vi "GEOM_CalcHeaders.vi"(8 "error in (no error)":errorcluster, 9 "modifiers":T2={"Binning"={"x"=1, "y"=1}, "sections"=[{"name"="", "header section"="", "comment"="", "value"=20, "binning?"=FALSE, "Where"=enum."predata", "add In"=enum."columns"}, {"name"="", "header section"="", "comment"="", "value"=64, "binning?"=FALSE, "Where"=enum."postdata", "add In"=enum."columns"}, {"name"="", "header section"="", "comment"="", "value"=14, "binning?"=FALSE, "Where"=enum."postdata", "add In"=enum."none"}]} {"Binning"."y" min=1; "Binning"."x" min=1}, 10 "FPAReadModes":T5[](array[typedef])=[{"name"="quad", "Amplifiers"=[{"number"=0, "type"=0, "rotated"=0, "fliped"=0, "FPAcoord"={"xstart"=1, "ystart"=1}, "Physical_size"={"columns"=1024, "rows"=1024}, "predata"={"columns"=20, "rows"=0}, "postdata"={"columns"=64, "rows"=0}, "Req ROIs"=[], "Corr ROI"=[], "Detnumber"=0, "ampID"="", "discard"=0}, {"number"=0, "type"=1, "rotated"=0, "fliped"=0, "FPAcoord"={"xstart"=1025, "ystart"=1}, "Physical_size"={"columns"=1024, "rows"=1024}, "predata"={"columns"=20, "rows"=0}, "postdata"={"columns"=64, "rows"=0}, "Req ROIs"=[], "Corr ROI"=[], "Detnumber"=0, "ampID"="", "discard"=0}, {"number"=0, "type"=2, "rotated"=0, "fliped"=0, "FPAcoord"={"xstart"=1, "ystart"=1025}, "Physical_size"={"columns"=1024, "rows"=1024}, "predata"={"columns"=20, "rows"=0}, "postdata"={"columns"=64, "rows"=0}, "Req ROIs"=[], "Corr ROI"=[], "Detnumber"=0, "ampID"="", "discard"=0}, {"number"=0, "type"=3, "rotated"=0, "fliped"=0, "FPAcoord"={"xstart"=1025, "ystart"=1025}, "Physical_size"={"columns"=1024, "rows"=1024}, "predata"={"columns"=20, "rows"=0}, "postdata"={"columns"=64, "rows"=0}, "Req ROIs"=[], "Corr ROI"=[], "Detnumber"=0, "ampID"="", "discard"=0}]}, {"name"="lowerleft", "Amplifiers"=[{"number"=0, "type"=0, "rotated"=0, "fliped"=0, "FPAcoord"={"xstart"=1, "ystart"=1}, "Physical_size"={"columns"=2048, "rows"=2048}, "predata"={"columns"=20, "rows"=0}, "postdata"={"columns"=64, "rows"=0}, "Req ROIs"=[], "Corr ROI"=[], "Detnumber"=0, "ampID"="", "discard"=0}]}] {"Amplifiers"."fliped" items=["none", "horizontal", "vertical"]; "Amplifiers"."type" items=["LL", "LR", "UL", "UR"]}, 11 "moddir":path=path "/kkk") -> (0 "error out":errorcluster)   [LabVIEW 2016]
uses:
  GEOM_FPAReadMode.ctl
  GEOM_Amplifier.ctl
  GEOM_AmpType.ctl
  GEOM_ROI.ctl
  GEOM_Coords.ctl
  GEOM_AmpModifiers.ctl
  GEOM_Binning.ctl
  GEOM_Moifier.ctl
  GEOM_ReadModeHeader.ctl
  GEOM_VAR_action.ctl
panel:
  in  "type specifier VI Refnum (for type only)":refnum<vi>
  in  "Empty Array 2":string[][](array[string])
  in  "Headers":T1
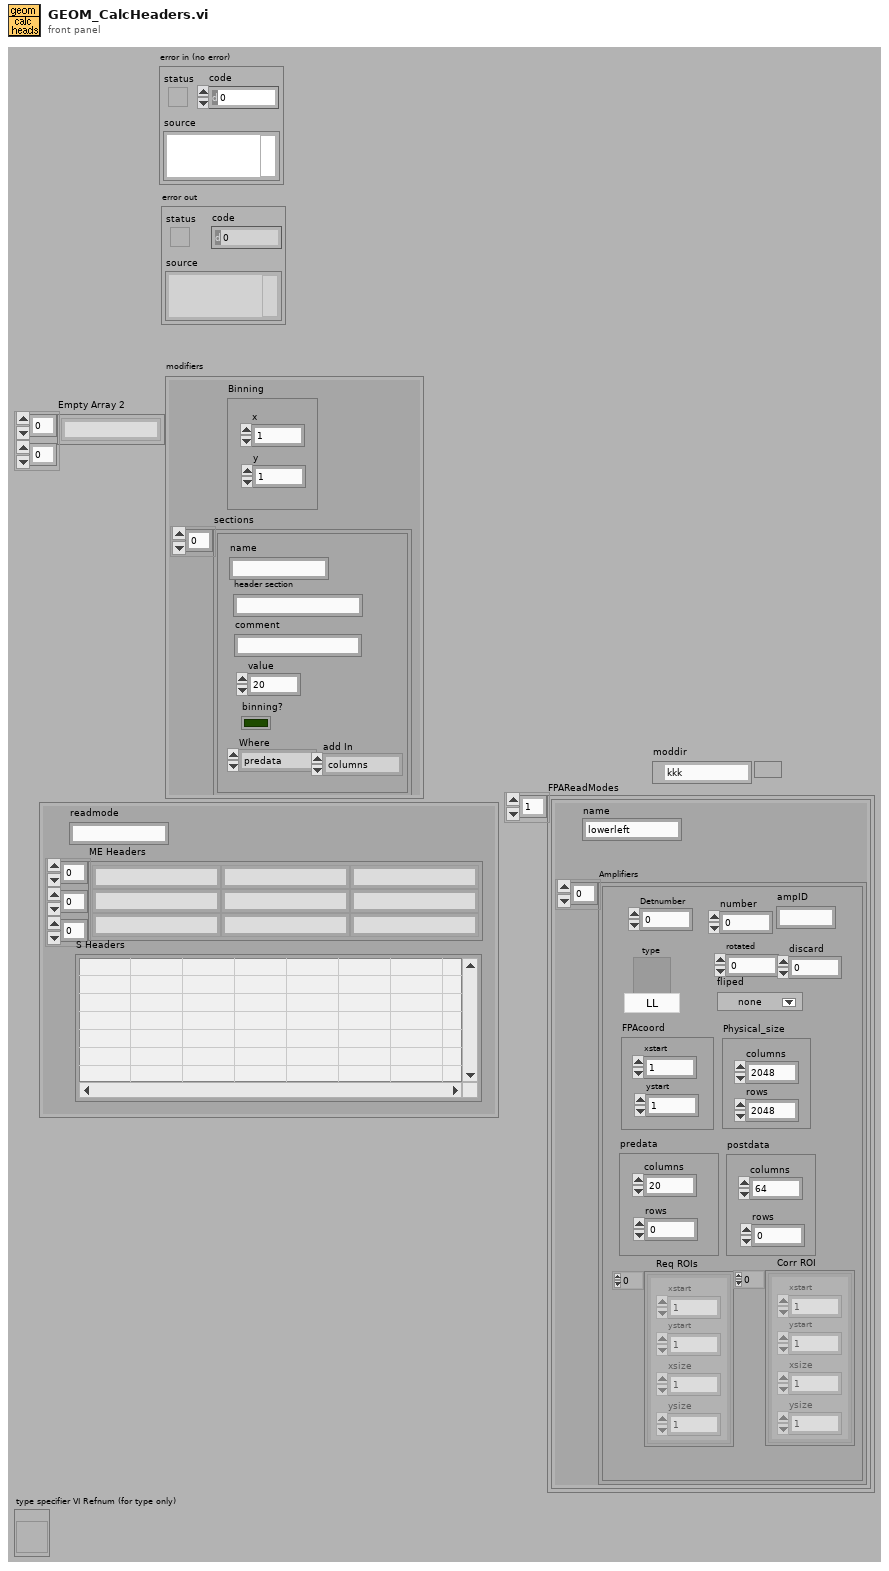
[diagram p1: front panel]
types:
  T1 = typedef "GEOM_ReadModeHeader.ctl" = cluster{"readmode":string, "ME Headers":string[][][], "S Headers":string[][]}
  T2 = typedef "GEOM_AmpModifiers.ctl" = cluster{"Binning":T3, "sections":T4[]}
  T3 = typedef "GEOM_Binning.ctl" = cluster{"x":u32, "y":u32}
  T4 = typedef "GEOM_Moifier.ctl" = cluster{"name":string, "header section":string, "comment":string, "value":i32, "binning?":bool, "Where":enum16{"predata", "postdata"}, "add In":enum16{"columns", "rows", "none"}}
  T5 = typedef "GEOM_FPAReadMode.ctl" = cluster{"name":string, "Amplifiers":T6[]}
  T6 = typedef "GEOM_Amplifier.ctl" = cluster{"number":i32, "type":T7, "rotated":i16, "fliped":u16, "FPAcoord":cluster{"xstart":i32, "ystart":i32}, "Physical_size":cluster{"columns":i32, "rows":i32}, "predata":cluster{"columns":i32, "rows":i32}, "postdata":cluster{"columns":i32, "rows":i32}, "Req ROIs":T8, "Corr ROI":T8, "Detnumber":i32, "ampID":string, "discard":i32}
  T7 = typedef "GEOM_AmpType.ctl" = u16
  T8 = typedef "GEOM_ROI.ctl" = T9[]
  T9 = typedef "GEOM_Coords.ctl" = cluster{"xstart":u32, "ystart":u32, "xsize":u32, "ysize":u32}
  T10 = typedef "GEOM_VAR_action.ctl" = enum16{"read", "write"}
  T11 = typedef "GEOM_CorrectedFPA.ctl" = cluster{"readmode":string, "amplifiers":cluster{"number":i32, "xstart":i32, "ystart":i32}[], "totxsize":i32, "totysize":i32, "maxxdim":i32, "maxydim":i32, "numxamps":i32, "numyamps":i32, "totxdata":i32, "totydata":i32, "xdataamp":i32, "ydataamp":i32, "totpixels":i32}
  T12 = typedef "GEOM_DetSummaryStruct.ctl" = cluster{"detxpos":i32, "detypos":i32, "cols":i32, "rows":i32, "nxamps":i32, "nyamps":i32, "number":i32, "discard":i32, "totcols":i32, "totrows":i32, "readmode":string}
  T13 = typedef "GEOM_HeaderModule.ctl" = cluster{"name":string, "Keys":string[][]}
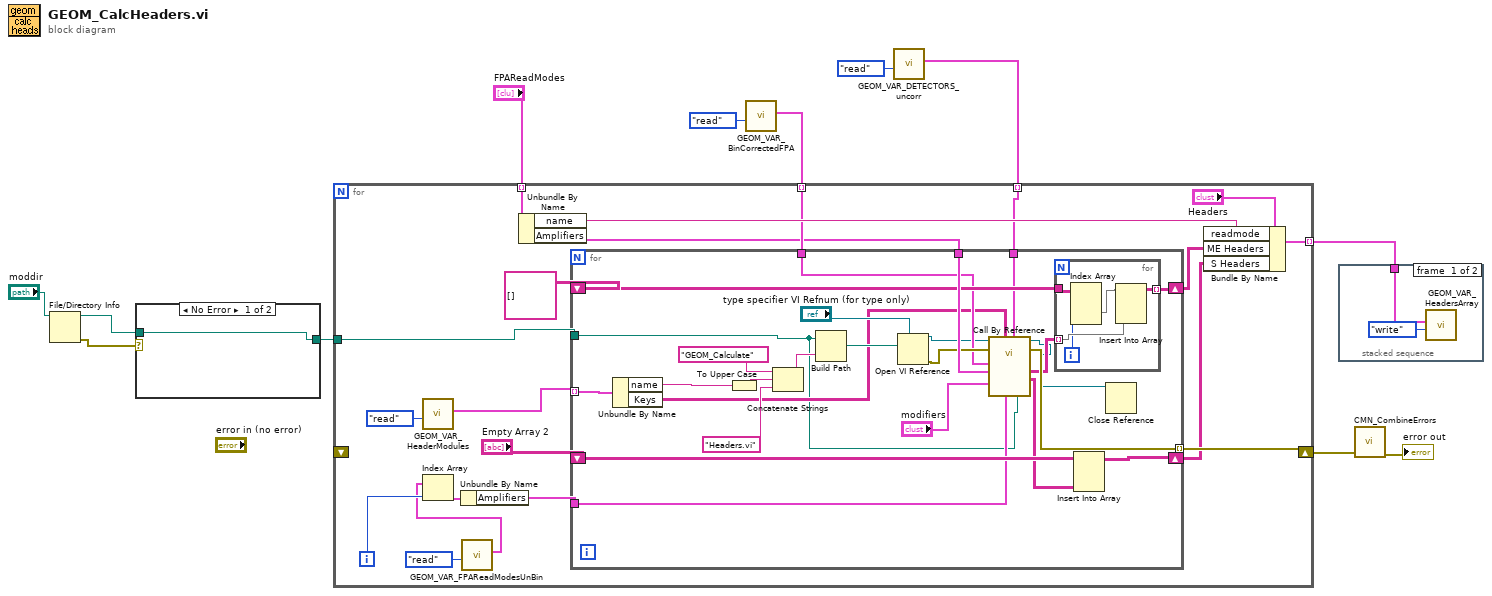
[diagram p0: block diagram]
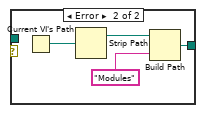
[diagram p2: hidden frame]
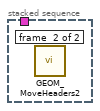
[diagram p3: hidden frame]
diagram:
  n1 = File/Directory Info(path="moddir") -> (path out=w3:path, error out=w5:errorcluster)  [unwired: 1 in, 5 out]
  n2 = case shown="No Error" w5 {
    tunnel: [w13 w14] -> w4
    tunnel: w3 -> [w13 _]
    frame No Error {
    }
    frame Error {
      n3 = Current VI's Path() -> (path=w15:path)
      n4 = Strip Path(path=w15) -> (stripped path=w16:path)  [unwired: 1 out]
      n5 = Build Path(base path=w16, name or relative path="Modules") -> (appended path=w14:path)
    }
  }
  n6 = call "GEOM_VAR_BinCorrectedFPA.vi"("Action"=GEOM_VAR_action."read") -> ("GEOM_BinCorrectedFPA out"=w7:T11[])  [unwired: 1 in, 9 out]
  n7 = call "GEOM_VAR_DETECTORS_uncorr.vi"("Action"=GEOM_VAR_action."read") -> ("det out"=w1:cluster{"name":string, "detectors":T12[]}[])  [unwired: 1 in, 9 out]
  n8 = for {
    tunnel: "FPAReadModes" -> [w37] mode=indexing
    tunnel: [w35] -> w10 mode=indexing
    shift-right: [w33] -> w12
    shift-left: _ -> [_]
    tunnel: w7 -> [w31] mode=indexing
    tunnel: w4 -> [w21]
    tunnel: w1 -> [w20] mode=indexing
    i -> [w26]
    n9 = call "GEOM_VAR_HeaderModules.vi"("Action"=GEOM_VAR_action."read") -> ("GEOM_HeaderModules out"=w23:T13[])  [unwired: 1 in, 9 out]
    n10 = call "GEOM_VAR_FPAReadModesUnBin.vi"("Action"=GEOM_VAR_action."read") -> ("GEOM_FPAReadModes out"=w18:T5[])  [unwired: 1 in, 9 out]
    n11 = Index Array(array=w18, index=w26) -> (element=w25:T5)
    n12 = Unbundle By Name(w25) -> ("Amplifiers"=w24:T6[])
    n13 = Unbundle By Name(w37) -> ("name"=w36:string, "Amplifiers"=w27:T6[])
    n14 = for {
      tunnel: w23 -> [w44] mode=indexing
      tunnel: w21 -> [w39]
      tunnel: w27 -> [w58]
      shift-right: [w49] -> w34
      shift-left: string[][][] [] -> [w50]
      tunnel: [w55] -> w33 mode=indexing
      tunnel: w31 -> [w47]
      shift-right: [w52] -> w29
      shift-left: "Empty Array 2" -> [w54]
      tunnel: w24 -> [w48]
      tunnel: w20 -> [w38]
      n15 = Unbundle By Name(w44) -> ("name"=w43:string, "Keys"=w41:string[][])
      n16 = To Upper Case(1:w43) -> (0:w42:string)
      n17 = Concatenate Strings("GEOM_Calculate" ("string"), w42, "Headers.vi" ("string")) -> (w61:string)
      n18 = Build Path(base path=w39, name or relative path=w61) -> (appended path=w60:path)
      n19 = Open VI Reference(type specifier VI Refnum (for type only)="type specifier VI Refnum (for type only)", vi path=w60) -> (vi reference=w45:refnum<vi>, error out=w56:errorcluster)  [unwired: 1 in, 3 out]
      n20 = call-by-ref "?"(reference=w45, error in=w56, "mpath"=w39, "detreadmodes"=w38, "ORIG Amplifiers"=w48, "args"=w41, "AmpModifiers"="modifiers", "Amplifiers"=w58, "Correctedamplifier"=w47) -> (reference out=w40:refnum<vi>, error out=w55:errorcluster, "S Headers out"=w53:string[][], "ME Headers out"=w51:string[][][])  [unwired: 3 in]
      n21 = for {
        tunnel: w51 -> [w67] mode=indexing
        tunnel: w50 -> [w65]
        tunnel: [w66] -> w49 mode=indexing
        i -> [w64]
        n22 = Index Array(array=w65, index (dim 0)=w64) -> (element=w63:string[][])  [unwired: 2 in]
        n23 = Insert Into Array(array=w63, new element=w67) -> (w66:string[][])  [unwired: 2 in]
      }
      n24 = Insert Into Array(array=w54, new element=w53) -> (w52:string[][])  [unwired: 2 in]
      n25 = Close Reference(reference=w40) -> ()  [unwired: 1 in, 1 out]
    }
    n26 = Bundle By Name(cluster="Headers", "readmode"=w36, "ME Headers"=w34, "S Headers"=w29) -> (w35:T1)
  }
  n27 = stacked-sequence {
    tunnel: w10 -> [w69 _]
    frame #0 {
      n28 = call "GEOM_VAR_HeadersArray.vi"("Action"=GEOM_VAR_action."write", "GEOM_HeadersArray"=w69) -> ()  [unwired: 10 out]
    }
    frame #1 {
      n29 = call "GEOM_MoveHeaders2.vi"() -> ()  [unwired: 12 out]
    }
  }
  n30 = call "CMN_CombineErrors.vi"("Errors"=w12) -> ("error out"=→"error out":errorcluster)  [unwired: 10 out]
